vi "setBurstCycles.vi"(8 "error in (no error)":errorcluster, 10 "NCycles":i32=-1, 11 "VISA resource name":refnum<visa-resource-name>) -> (0 "error out":errorcluster, 3 "VISA resource name out":refnum<visa-resource-name>)   [LabVIEW 2023, in "Keysight-33500B.lvlib"]
doc: "<b>Author:</b> Wolfgang\n<b>Description:</b>\nSets the number of cycles to be output per burst (triggered burst mode only)."
uses:
  Keysight-33500B.lvlib
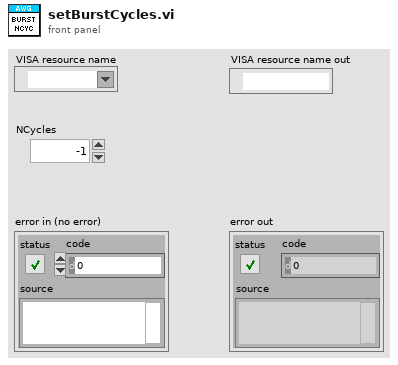
[diagram p1: front panel]
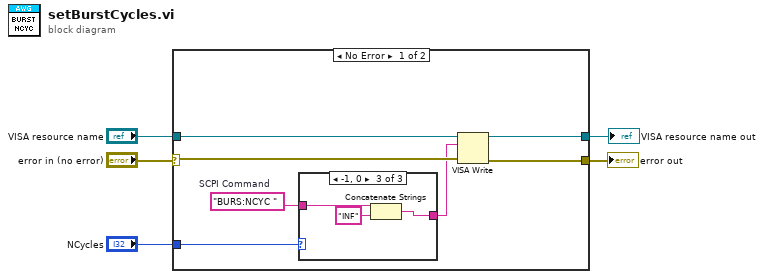
[diagram p0: block diagram]
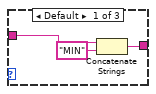
[diagram p2: hidden frame]
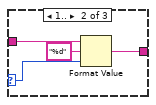
[diagram p3: hidden frame]
diagram:
  n1 = case shown="No Error" "error in (no error)" {
    selector: "error in (no error)" -> [w9 w24]
    tunnel: [w11 w23] -> w5
    tunnel: [w12 w24] -> w3
    tunnel: "VISA resource name" -> [w10 w23]
    tunnel: "NCycles" -> [w8 _]
    frame No Error {
      w7 = "BURS:NCYC "  # SCPI Command
      n2 = case shown="-1, 0" w8 {
        selector: w8 -> [_ w17 _]
        tunnel: w7 -> [w15 w18 w21]
        tunnel: [w14 w19 w22] -> w6
        frame Default {
          n3 = Concatenate Strings(w15, "MIN" ("string")) -> (w14:string)
        }
        frame 1.. {
          n4 = Format Value(string ("")=w18, format string="%d", value (0)=w17) -> (output string=w19:string)
        }
        frame -1, 0 {
          n5 = Concatenate Strings(w21, "INF" ("string")) -> (w22:string)
        }
      }
      n6 = VISA Write(VISA resource name=w10, write buffer=w6, error in (no error)=w9) -> (VISA resource name out=w11:refnum<visa-resource-name>, error out=w12:errorcluster)  [unwired: 1 out]
    }
    frame Error {
    }
  }
  "VISA resource name out" <- w5
  "error out" <- w3
